vi "Swap_TimeStamp[].vi"(4 "Swap(T)":bool=TRUE, 6 "b":timestamp[](array[timestamp]), 7 "a":timestamp[](array[timestamp])) -> (1 "b":timestamp[](array[timestamp]), 2 "a":timestamp[](array[timestamp]))   [LabVIEW 2012]
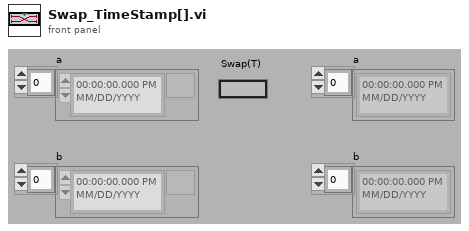
[diagram p1: front panel]
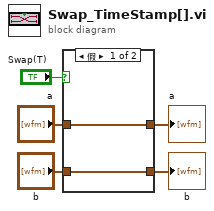
[diagram p0: block diagram]
diagram:
  n1 = case shown="假" "Swap(T)" {
    tunnel: "a" -> [w7 w9]
    tunnel: "b" -> [w6 w8]
    tunnel: [w7 w8] -> w2
    tunnel: [w6 w9] -> w1
    frame False {
    }
    frame True {
    }
  }
  "a" <- w2
  "b" <- w1
